vi "new shift odd lines by.vi"(6 "max pix shift":i32=150, 7 "shift odd lines by":i32, 8 "calculate shited frame":bool, 11 "pixel array in (x is first dimension)":dbl[][](array[numeric])) -> (2 "squared difference":dbl, 3 "shifted frame out (x is first dimension)":dbl[][](array[numeric]))   [LabVIEW 2012]
doc: "SciScan 1.2 160622"
panel:
  out "corrected 4":T1(plugin-control)
  out "size(s) 12":i32
  out "size(s) 11":i32
  out "size(s) 10":i32[](array[numeric])
  out "corrected":T1(plugin-control)
  out "size(s) 9":i32[](array[numeric])
  out "size(s) 8":i32[](array[numeric])
  out "size(s) 7":i32[](array[numeric])
  out "Array 2":dbl[][](array[numeric])
  out "Array":dbl[][](array[numeric])
  out "size(s) 6":i32[](array[numeric])
  out "size(s) 5":i32[](array[numeric])
  out "size(s) 4":i32
  out "corrected 3":T1(plugin-control)
  out "size(s)":i32[](array[numeric])
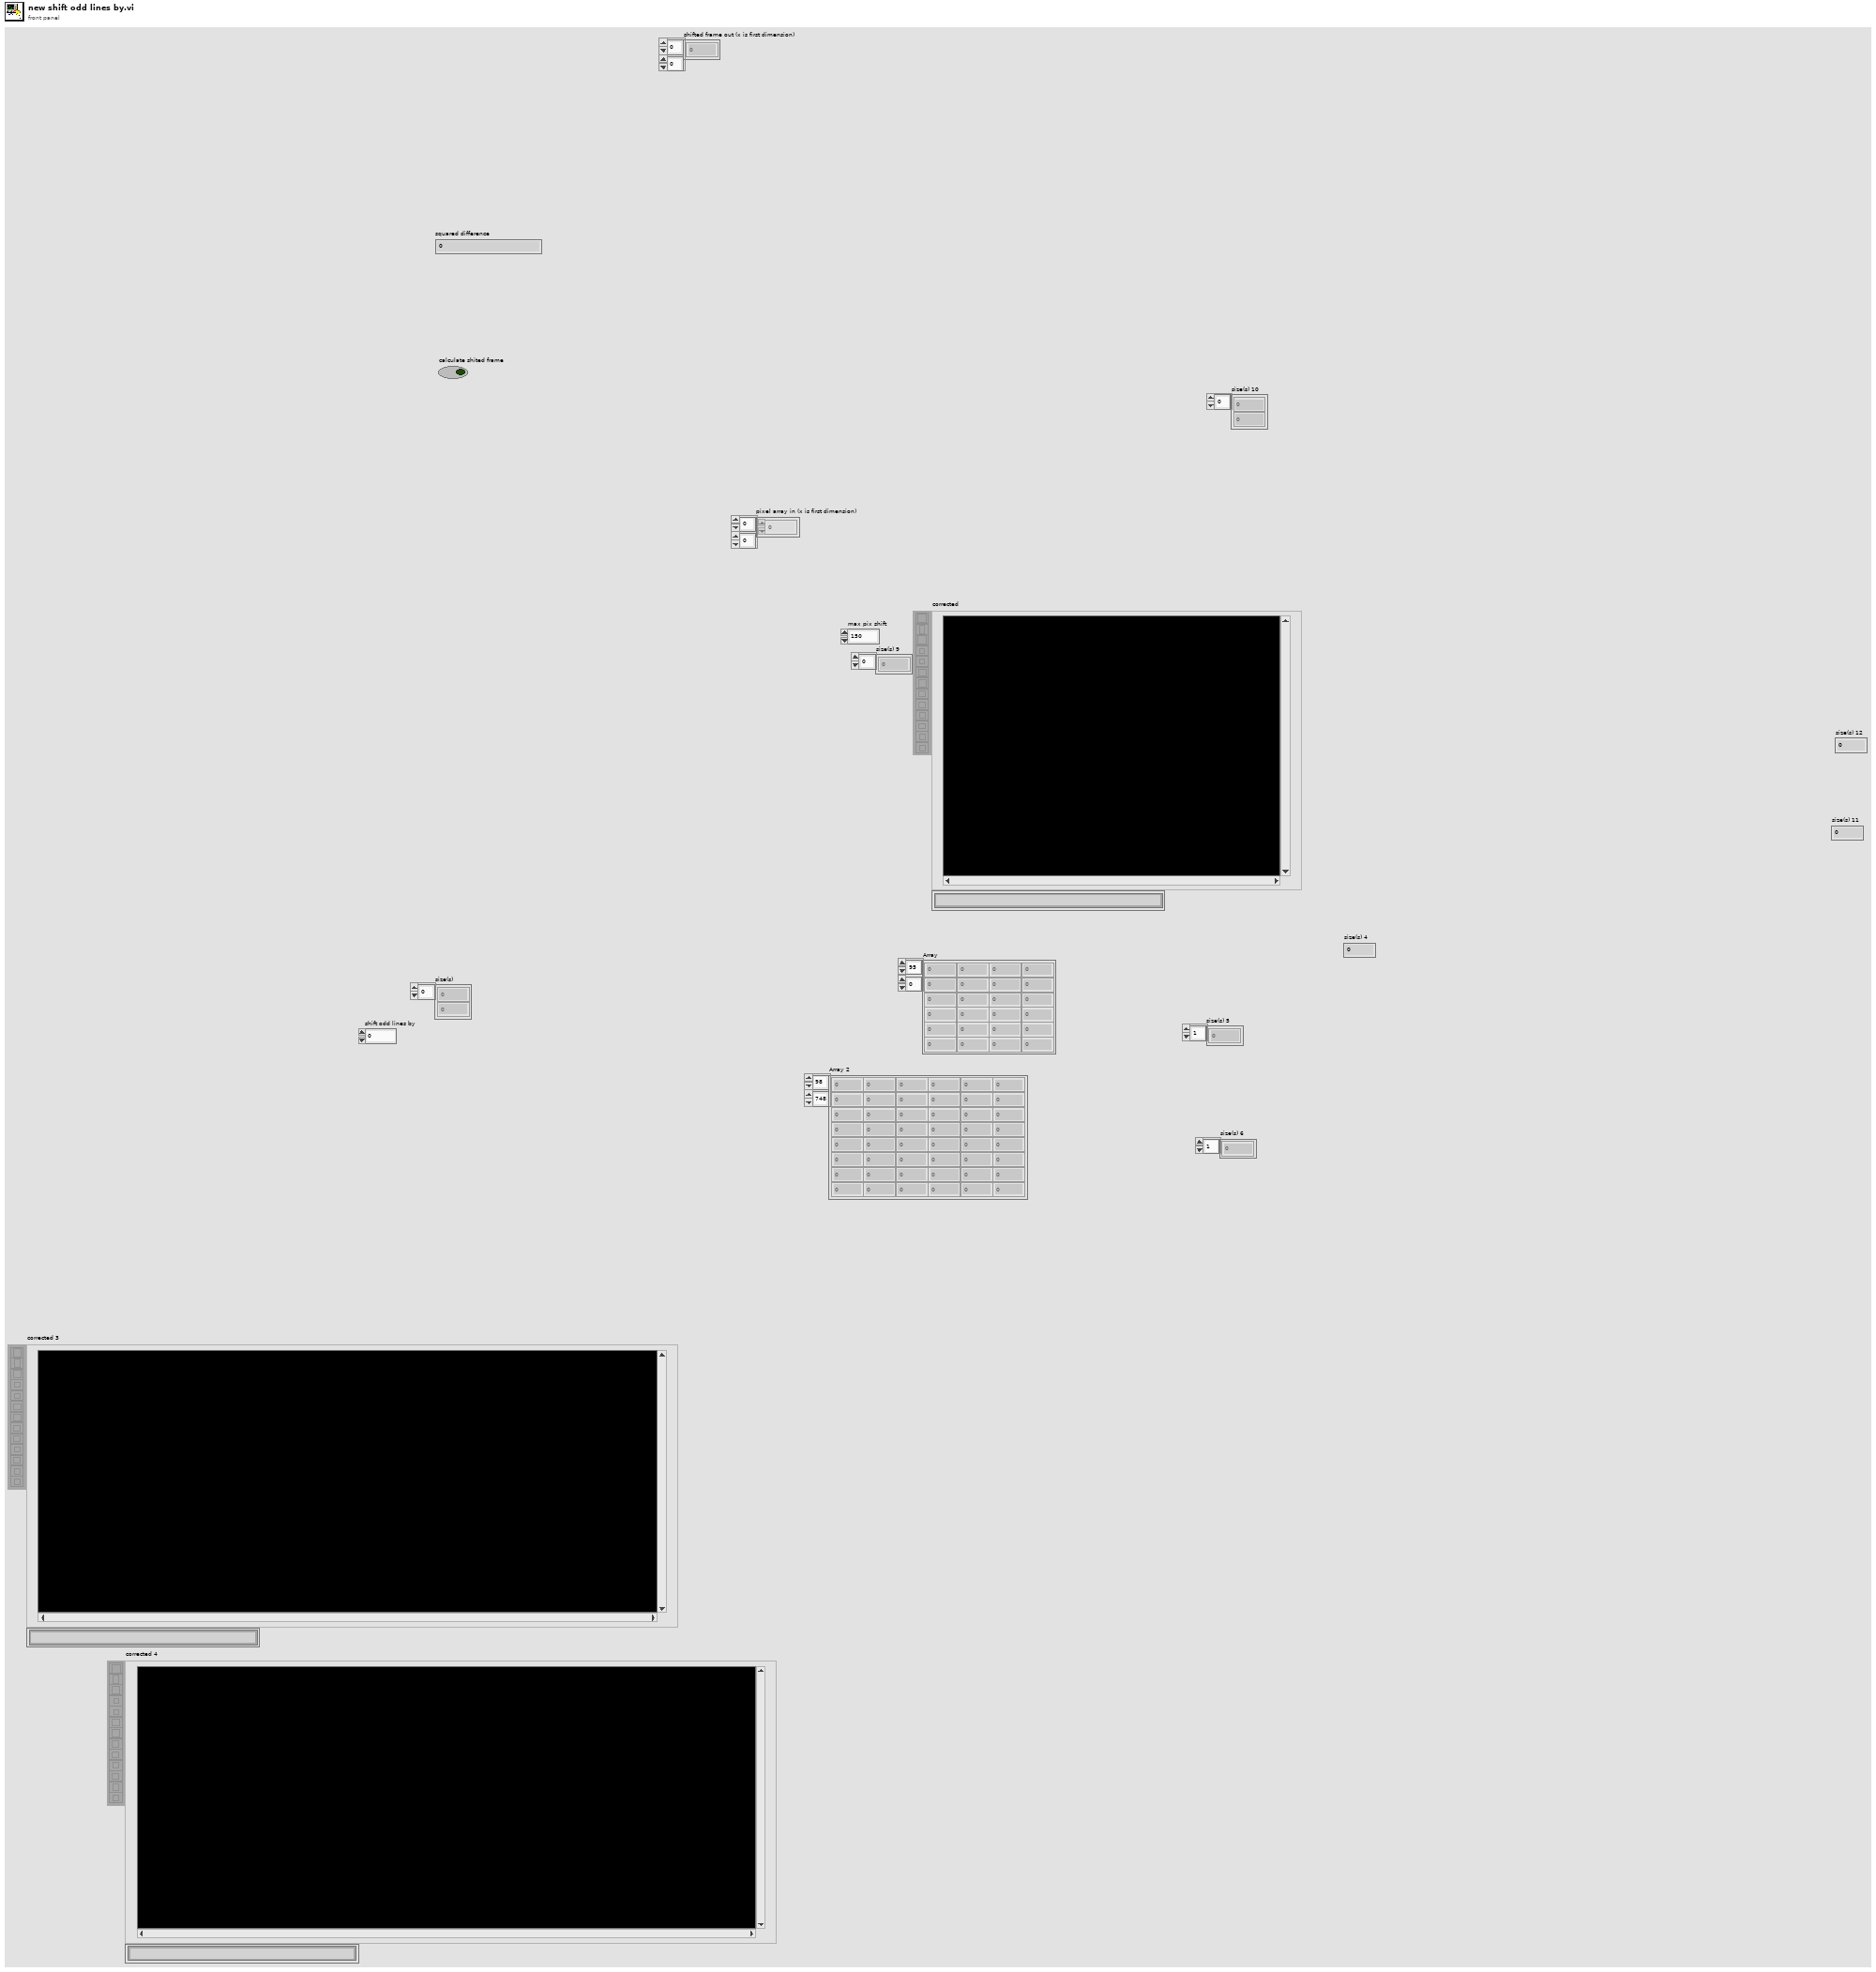
[diagram p1: front panel]
types:
  T1 = typedef "IMAQ Image.ctl" = refnum<image>
  T2 = typedef "Image Type" = u32
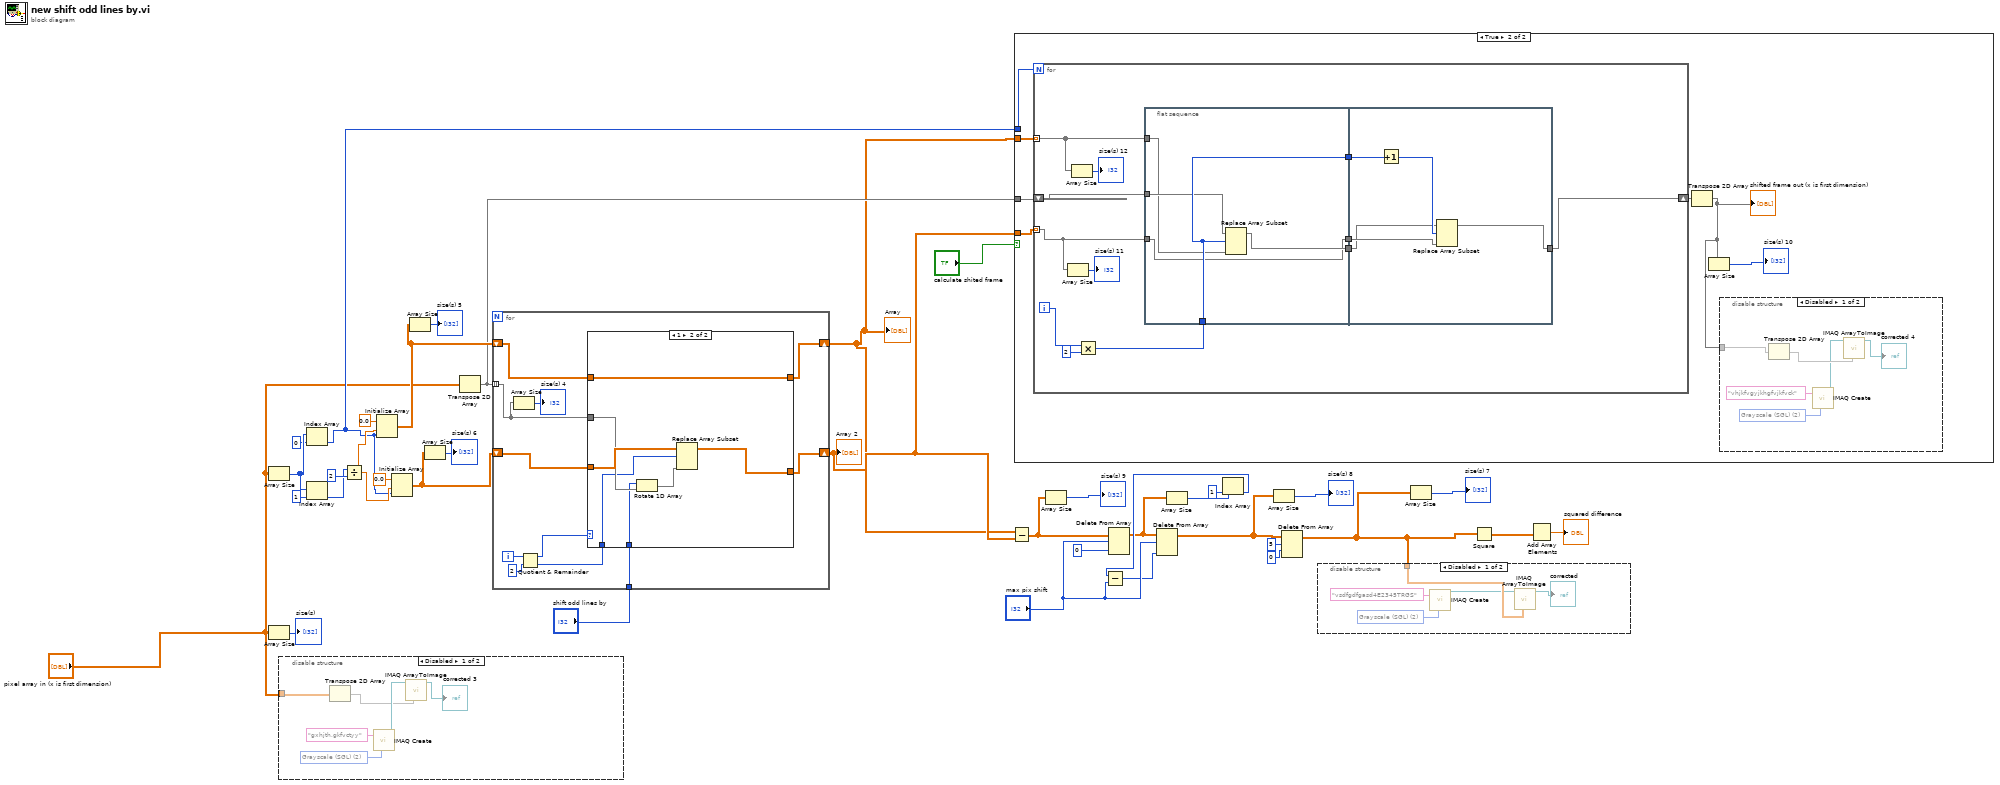
[diagram p0: block diagram]
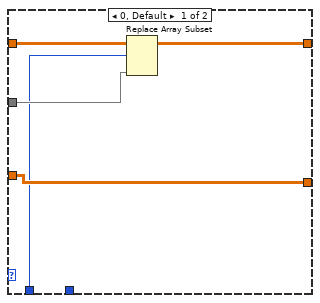
[diagram p6: hidden frame]
diagram:
  n1 = Array Size(array="pixel array in (x is first dimension)") -> (size(s)=w31:i32[])
  n2 = Array Size(array="pixel array in (x is first dimension)") -> (size(s)=→"size(s)":i32[])
  n3 = disable-structure shown="Disabled" {
    disable-tunnel: "pixel array in (x is first dimension)" -> [w39 _]
    frame Disabled {
      w40 = T2 2 items=["Grayscale (U8)", "Grayscale (I16)", "Grayscale (SGL)", "Complex (CSG)", "RGB (U32)", "HSL (U32)", "RGB (U64)", "Grayscale (U16)"] ("Image Type")
      n4 = Transpose 2D Array(2D array=w39) -> (transposed array=w38:dbl[][])
      n5 = call "IMAQ Create"("Image Name"="gxhjth,gkfvctyy", "Image Type"=w40) -> ("New Image"=w42:T1)  [unwired: 3 in, 1 out]
      n6 = call "IMAQ ArrayToImage"("Image Pixels (Float)"=w38, "Image"=w42) -> ("Image Out"=→"corrected 3":T1)  [unwired: 8 in, 1 out]
    }
    frame Enabled {
    }
  }
  n7 = Index Array(array=w31, index=0) -> (element=w3:i32)
  n8 = Index Array(array=w31, index=1) -> (element=w32:i32)
  n9 = Divide(x=w32, y=2) -> (x/y=w36:dbl)
  n10 = Initialize Array(0.0 ("element"), w36, w3) -> (w26:dbl[][])
  n11 = Initialize Array(0.0 ("element"), w36, w3) -> (w24:dbl[][])
  n12 = Array Size(array=w26) -> (size(s)=→"size(s) 5":i32[])
  n13 = Array Size(array=w24) -> (size(s)=→"size(s) 6":i32[])
  n14 = Transpose 2D Array(2D array="pixel array in (x is first dimension)") -> (transposed array=w5:dbl[][])
  n15 = for {
    tunnel: w5 -> [w45] mode=indexing
    shift-right: [w50] -> w4
    shift-left: w26 -> [w51]
    shift-right: [w47] -> w6
    shift-left: w24 -> [w48]
    tunnel: "shift odd lines by" -> [w46]
    i -> [w54]
    n16 = Array Size(array=w45) -> (size(s)=→"size(s) 4":i32)
    n17 = Quotient & Remainder(x=w54, y=2) -> (x-y*floor(x/y)=w52:i32, floor(x/y)=w49:i32)
    n18 = case shown="1" w52 {
      tunnel: w45 -> [w57 w65]
      tunnel: w51 -> [w59 w62]
      tunnel: [w58 w62] -> w50
      tunnel: w49 -> [w55 w60]
      tunnel: w48 -> [w56 w66]
      tunnel: [w56 w63] -> w47
      tunnel: w46 -> [_ w61]
      frame 0, Default {
        n19 = Replace Array Subset(array=w59, new element=w57, index (row)=w55) -> (w58:dbl[][])  [unwired: 1 in]
      }
      frame 1 {
        n20 = Rotate 1D Array(1:w65, 2:w61) -> (0:w64:dbl[])
        n21 = Replace Array Subset(array=w66, new element=w64, index (row)=w60) -> (w63:dbl[][])  [unwired: 1 in]
      }
    }
  }
  "Array" <- w4
  "Array 2" <- w6
  n22 = Subtract(x=w4, y=w6) -> (x-y=w15:dbl[][])
  n23 = case shown="True" "calculate shited frame" {
    tunnel: w6 -> [_ w73]
    tunnel: w5 -> [_ w72]
    tunnel: w4 -> [_ w71]
    tunnel: w3 -> [_ w70]
    frame False {
    }
    frame True {
      n24 = for {
        N: w70 -> [_]
        shift-right: [w89] -> w68
        shift-left: w72 -> [w91]
        tunnel: w71 -> [w80] mode=indexing
        tunnel: w73 -> [w82] mode=indexing
        i -> [w90]
        n25 = Array Size(array=w82) -> (size(s)=→"size(s) 11":i32)
        n26 = Array Size(array=w80) -> (size(s)=→"size(s) 12":i32)
        n27 = Multiply(x=w90, y=2) -> (x*y=w88:i32)
        n28 = flat-sequence {
          tunnel: w91 -> [w95]
          tunnel: [w93] -> w86
          tunnel: w82 -> [w92]
          tunnel: [w92] -> w85
          tunnel: w88 -> [w96]
          tunnel: [w96] -> w84
          tunnel: w80 -> [w94]
          tunnel: [w98] -> w89
          tunnel: w86 -> [w97]
          tunnel: w85 -> [w101]
          tunnel: w84 -> [w100]
          frame #0 {
            n29 = Replace Array Subset(array=w95, new element=w94, index (row)=w96) -> (w93:dbl[][])  [unwired: 1 in]
          }
          frame #1 {
            n30 = Increment(x=w100) -> (x+1=w99:i32)
            n31 = Replace Array Subset(array=w97, new element=w101, index (row)=w99) -> (w98:dbl[][])  [unwired: 1 in]
          }
        }
      }
      n32 = Transpose 2D Array(2D array=w68) -> (transposed array=w67:dbl[][])
      "shifted frame out (x is first dimension)" <- w67
      n33 = Array Size(array=w67) -> (size(s)=→"size(s) 10":i32[])
      n34 = disable-structure shown="Disabled" {
        disable-tunnel: w67 -> [w74 _]
        frame Disabled {
          w78 = T2 2 items=["Grayscale (U8)", "Grayscale (I16)", "Grayscale (SGL)", "Complex (CSG)", "RGB (U32)", "HSL (U32)", "RGB (U64)", "Grayscale (U16)"] ("Image Type")
          n35 = Transpose 2D Array(2D array=w74) -> (transposed array=w79:dbl[][])
          n36 = call "IMAQ Create"("Image Name"="vhjkfvgyjkhgfvjkfvck", "Image Type"=w78) -> ("New Image"=w76:T1)  [unwired: 3 in, 1 out]
          n37 = call "IMAQ ArrayToImage"("Image Pixels (Float)"=w79, "Image"=w76) -> ("Image Out"=→"corrected 4":T1)  [unwired: 8 in, 1 out]
        }
        frame Enabled {
        }
      }
    }
  }
  n38 = Array Size(array=w15) -> (size(s)=→"size(s) 9":i32[])
  n39 = Delete From Array(array=w15, length="max pix shift", index (col)=0 ("index (row)")) -> (array with subset deleted=w18:dbl[][])  [unwired: 1 in, 1 out]
  n40 = Array Size(array=w18) -> (size(s)=w21:i32[])
  n41 = Index Array(array=w21, index=1) -> (element=w19:i32)
  n42 = Subtract(x=w19, y="max pix shift") -> (x-y=w8:i32)
  n43 = Delete From Array(array=w18, length="max pix shift", index (col)=w8) -> (array with subset deleted=w12:dbl[][])  [unwired: 1 in, 1 out]
  n44 = Array Size(array=w12) -> (size(s)=→"size(s) 8":i32[])
  n45 = Delete From Array(array=w12, length=5, index (row)=0) -> (array with subset deleted=w10:dbl[][])  [unwired: 1 in, 1 out]
  n46 = disable-structure shown="Disabled" {
    disable-tunnel: w10 -> [w106 _]
    frame Disabled {
      w105 = T2 2 items=["Grayscale (U8)", "Grayscale (I16)", "Grayscale (SGL)", "Complex (CSG)", "RGB (U32)", "HSL (U32)", "RGB (U64)", "Grayscale (U16)"] ("Image Type")
      n47 = call "IMAQ Create"("Image Name"="vsdfgdfgasd4E2345TRGS", "Image Type"=w105) -> ("New Image"=w103:T1)  [unwired: 3 in, 1 out]
      n48 = call "IMAQ ArrayToImage"("Image Pixels (Float)"=w106, "Image"=w103) -> ("Image Out"=→"corrected":T1)  [unwired: 8 in, 1 out]
    }
    frame Enabled {
    }
  }
  n49 = Array Size(array=w10) -> (size(s)=→"size(s) 7":i32[])
  n50 = Square(x=w10) -> (x^2=w23:dbl[][])
  n51 = Add Array Elements(numeric array=w23) -> (sum=→"squared difference":dbl)
